vi "QAM Demodulation.vi"(9 "pulse shaping filter (none)":T1(ring)) -> (0 "QAM synchronization parameters":T3, 1 "matched filter coefficients":dbl[](array[numeric]), 2 "QAM system parameters":T2, 3 "output bit stream":i8[](array[numeric]))   [LabVIEW 2026]
uses:
  <vilib>/addons/Modulation/Digital/General/MT Generate Bits (Galois, PN Order).vi
  <vilib>/addons/Modulation/Digital/Support/Common/Validators/mod_Generate Bits Validate.vi
  <vilib>/addons/Modulation/Analog/support/mod_Set Error Source.vi
  <vilib>/addons/Modulation/Digital/General/subVIs/mod_Generate Bits PN Sequence.vi
  <vilib>/addons/Modulation/Digital/General/MT Generate QAM System Parameters(M).vi
  <vilib>/addons/Modulation/Digital/General/MT Generate QAM Synchronization Parameters (bit array).vi
  <vilib>/addons/Modulation/Digital/Support/Common/Validators/mod_Generate Filter Coefficients Validate.vi
  <vilib>/addons/Modulation/Digital/General/subVIs/mod_Generate Filter Coefficients.vi
  <vilib>/addons/Modulation/niDMT.lvlib
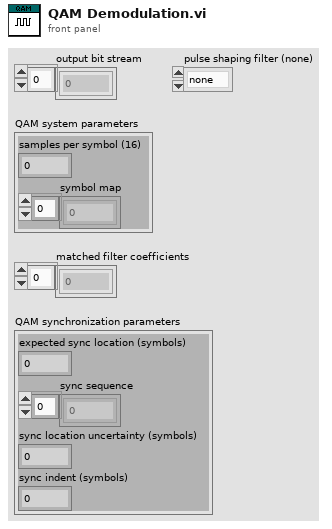
[diagram p1: front panel]
types:
  T1 = enum16{"none", "Raised Cosine", "Root Raised Cos", "Gaussian"}
  T2 = cluster{"samples per symbol (16)":i32, "symbol map":cdb[]}
  T3 = cluster{"expected sync location (symbols)":i32, "sync sequence":cdb[], "sync location uncertainty (symbols)":i32, "sync indent (symbols)":i32}
  T4 = enum16{"FSK", "PSK", "QAM", "MSK", "PAM", "ASK", "CPM"}
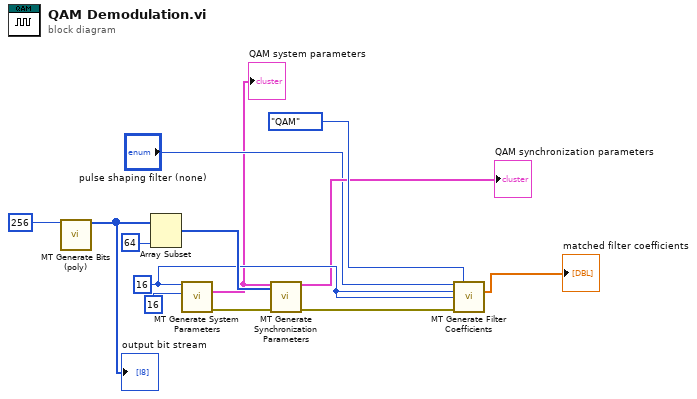
[diagram p0: block diagram]
diagram:
  w11 = 16 ("samples per symbol (16)")
  n1 = call-poly <vilib>:"MT Generate Bits (poly).vi"("total bits (128)"=256) -> ("output bit stream"=w13:i8[])  [unwired: 12 in, 2 out]
  "output bit stream" <- w13
  n2 = Array Subset(array=w13, length=64) -> (w12:i8[])  [unwired: 1 in]
  n3 = call-poly <vilib>:"MT Generate System Parameters.vi"("samples per symbol (16)"=w11, "M-QAM (16)"=16) -> ("QAM system parameters"=w5:T2, "error out"=w4:errorcluster)  [unwired: 11 in, 1 out]
  "QAM system parameters" <- w5
  n4 = call-poly <vilib>:"MT Generate Synchronization Parameters.vi"("QAM system parameters"=w5, "sync bits"=w12, "error in (no error)"=w4) -> ("QAM synchronization parameters"=→"QAM synchronization parameters":T3, "error out"=w3:errorcluster)  [unwired: 11 in]
  n5 = call <vilib>:"MT Generate Filter Coefficients.vi"("pulse shaping filter (none)"="pulse shaping filter (none)", "modulation type"=T4."QAM", "pulse shaping samples per symbol (16)"=w11, "matched samples per symbol (16)"=w11, "error in (no error)"=w3) -> ("matched filter coefficients"=→"matched filter coefficients":dbl[])  [unwired: 8 in, 2 out]
